vi "PUBSUB-CHANNELS.vi"(0 "refnum in":refnum<vi>, 5 "Use Pattern ?":bool, 7 "Pattern":string, 11 "error in":errorcluster) -> (4 "refnum out":refnum<vi>, 6 "Data":T1, 15 "error out":errorcluster)   [LabVIEW 2023]
uses:
  SubVIs/Controls/redis-data.ctl
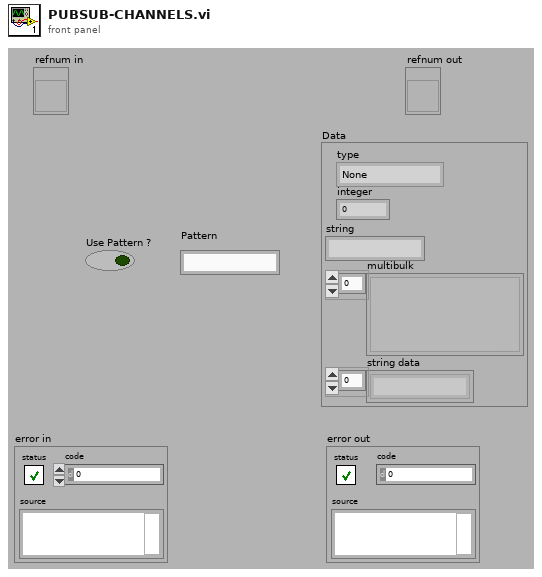
[diagram p1: front panel]
types:
  T1 = typedef "redis-data.ctl" = cluster{"type":enum16{"None", "Error", "Status", "Nil", "Integer", "String", "Multibulk"}, "integer":i64, "string":string, "multibulk":variant[], "string data":string[]}
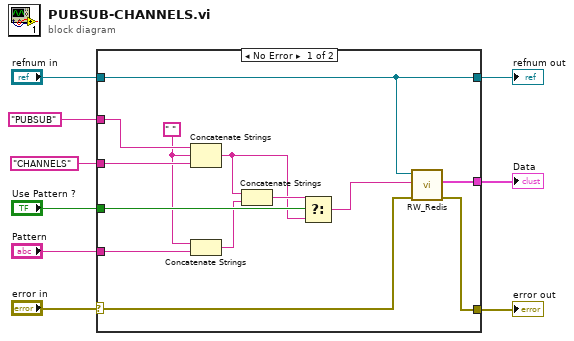
[diagram p0: block diagram]
diagram:
  n1 = case shown="No Error" "error in" {
    selector: "error in" -> [w21 w24]
    tunnel: "CHANNELS" -> [w18 _]
    tunnel: "PUBSUB" -> [w22 _]
    tunnel: "refnum in" -> [w12 w23]
    tunnel: [w20 w24] -> w7
    tunnel: [w19 _] -> w2
    tunnel: "Pattern" -> [w10 _]
    tunnel: "Use Pattern ?" -> [w17 _]
    tunnel: [w12 w23] -> w4
    frame No Error {
      w16 = " "
      n2 = Concatenate Strings(w22, w16, w18) -> (w14:string)
      n3 = Concatenate Strings(w16, w10) -> (w13:string)
      n4 = Concatenate Strings(w14, w13) -> (w15:string)
      n5 = Select(t=w15, s=w17, f=w14) -> (s? t:f=w11:string)
      n6 = call "RW_Redis.vi"("error in"=w21, "command"=w11, "TCP session in"=w12) -> ("error out"=w20:errorcluster, "Data"=w19:T1)  [unwired: 6 in, 1 out]
    }
    frame Error {
    }
  }
  "error out" <- w7
  "Data" <- w2
  "refnum out" <- w4
